vi "Input_Commands_TipperV2.vi"(11 "All Joysticks":T2) -> (3 "Tipper Command Inputs":T1)   [LabVIEW 2011]
uses:
  Input_All_Joysticks.ctl
  Input_Single_Joystick.ctl
  <vilib>/Rock Robotics/WPI/Joystick/WPI_JoystickButtonState.ctl
  Inputs_Tipper.ctl
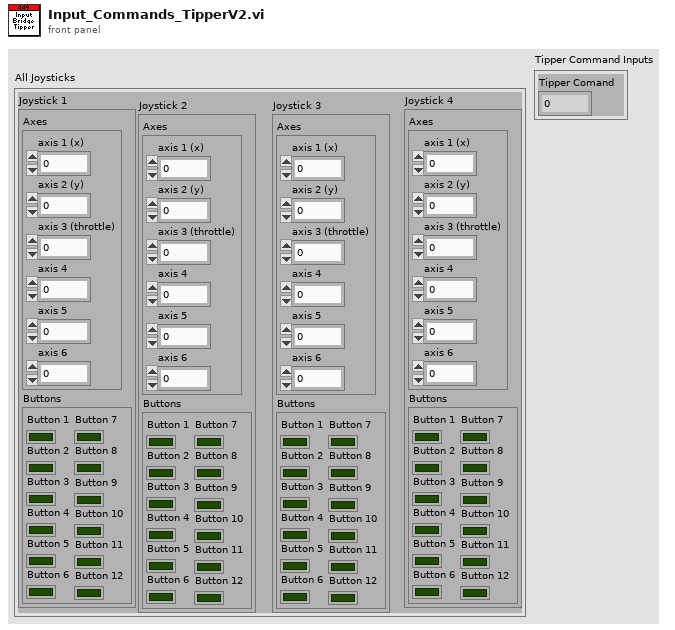
[diagram p1: front panel]
types:
  T1 = typedef "Inputs_Tipper.ctl" = cluster{"Tipper Comand":dbl}
  T2 = typedef "Input_All_Joysticks.ctl" = cluster{"Joystick 1":T3, "Joystick 2":T3, "Joystick 3":T3, "Joystick 4":T3}
  T3 = typedef "Input_Single_Joystick.ctl" = cluster{"Axes":cluster{"axis 1 (x)":dbl, "axis 2 (y)":dbl, "axis 3 (throttle)":dbl, "axis 4":dbl, "axis 5":dbl, "axis 6":dbl}, "Buttons":T4}
  T4 = typedef "WPI_JoystickButtonState.ctl" = cluster{"Button 1":bool, "Button 2":bool, "Button 3":bool, "Button 4":bool, "Button 5":bool, "Button 6":bool, "Button 7":bool, "Button 8":bool, "Button 9":bool, "Button 10":bool, "Button 11":bool, "Button 12":bool}
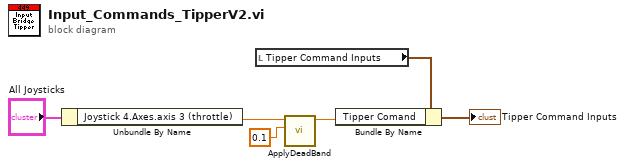
[diagram p0: block diagram]
diagram:
  n1 = Unbundle By Name("All Joysticks") -> ("Joystick 4.Axes.axis 3 (throttle)"=w4:dbl)
  n2 = local read "Tipper Command Inputs"() -> (w5:T1)
  n3 = call "ApplyDeadBand.vi"("Deadband"=0.1, "Input"=w4) -> ("Input with deadband"=w3:dbl)  [unwired: 9 in]
  n4 = Bundle By Name(cluster=w5, "Tipper Comand"=w3) -> (→"Tipper Command Inputs":T1)
